vi "rad_Convert FPGA Properties to Item Strings.vi"(7 "MCListbox Refnum":refnum<vi>, 11 "FPGA Properties":T1) -> (3 "Item Names":string[](array[string]))   [LabVIEW 2013]
uses:
  TypeDefs/rad_FPGA Flash Properties.ctl
  <vilib>/Utility/miscctls.llb/LVRowAndColumnTypeDef.ctl
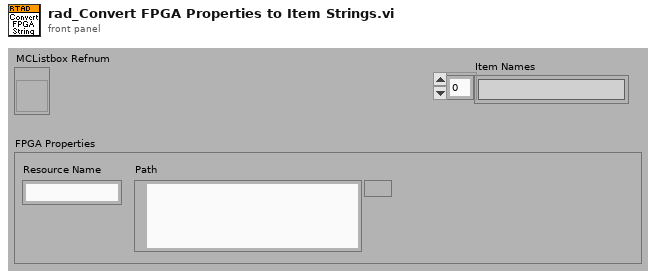
[diagram p1: front panel]
types:
  T1 = typedef "rad_FPGA Flash Properties.ctl" = cluster{"Resource Name":string, "Path":path}
  T2 = typedef "LVRowAndColumnTypeDef.ctl" = cluster{"Row":i32, "Column":i32}
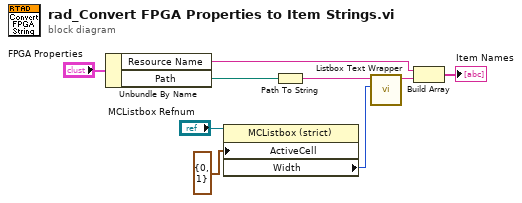
[diagram p0: block diagram]
diagram:
  n1 = Unbundle By Name("FPGA Properties") -> ("Resource Name"=w4:string, "Path"=w3:path)
  n2 = property on="Property Node" class="MCListbox (strict)"(reference="MCListbox Refnum", "ActiveCell"=T2 {"Row"=0, "Column"=1} ("Active Cell:Active Cell")) -> ("Width"=w8:u32)  [unwired: 1 in, 2 out]
  n3 = Path To String(path=w3) -> (string=w7:string)
  n4 = call "Listbox Text Wrapper.vi"("Size:Width"=w8, "Input Text"=w7) -> ("Wrapped Text"=w9:string)  [unwired: 9 in]
  n5 = Build Array(w4, w9) -> (→"Item Names":string[])
